vi "FPGA Main.vi"(8 "Read":bool) -> (4 "Element in Buffer":u32[](array[numeric])=[189, 189, 189, 189])   [LabVIEW 2011]
uses:
  <vilib>/rvi/eio/common/nirviEmuTemplateMethod_errors.vi
  <vilib>/rvi/DataTransferAndStorage/Container/Common/niFpgaContainerExecOnDevCompGetState.vi
  <vilib>/rvi/FIFO/Fifo_Resource/nirvififoEmulationSetSize.vi
  <vilib>/rvi/DataTransferAndStorage/Container/Common/niFpgaContainerGetUniqueNameForEmu.vi
  <vilib>/rvi/interface/RandomDataEmulation/nirviRandomDataFPGAFIFO.vi
  <vilib>/rvi/interface/RandomDataEmulation/niFpgaRandomDataHandleErrors.vi
  <vilib>/rvi/eio/common/nirviEmuReportErrorAndStop.vi
  Global_Read.vi
  <vilib>/eio/EIONode/EIONode.xnode
  <vilib>/rvi/DataTransferAndStorage/Container/XNode/niFpgaContainer.xnode
  <vilib>/rvi/FIFO/Fifo_Resource/niFpgaFifoEmulationRefIn.vi
panel:
  out "Beat":bool=TRUE
  in  "Edge":bool
  in  "Buffer#4":i32
  in  "Buffer#3":i32
  in  "Buffer#2":i32
  in  "Buffer#1":i32
  in  "Port Settings - 4 Chan":T1(array[cluster])=[{"Data Bit(8)"=8, "Stop Bit"=1, "Baud Rate"=9600, "Invert Polarity?"=TRUE, " Mode"=FALSE}, {"Data Bit(8)"=0, "Stop Bit"=0, "Baud Rate"=0, "Invert Polarity?"=FALSE, " Mode"=FALSE}, {"Data Bit(8)"=0, "Stop Bit"=0, "Baud Rate"=0, "Invert Polarity?"=FALSE, " Mode"=FALSE}, {"Data Bit(8)"=0, "Stop Bit"=0, "Baud Rate"=0, "Invert Polarity?"=FALSE, " Mode"=FALSE}] {"Stop Bit" items=["1.0"=10, "1.5"=15, "2.0"=20]}
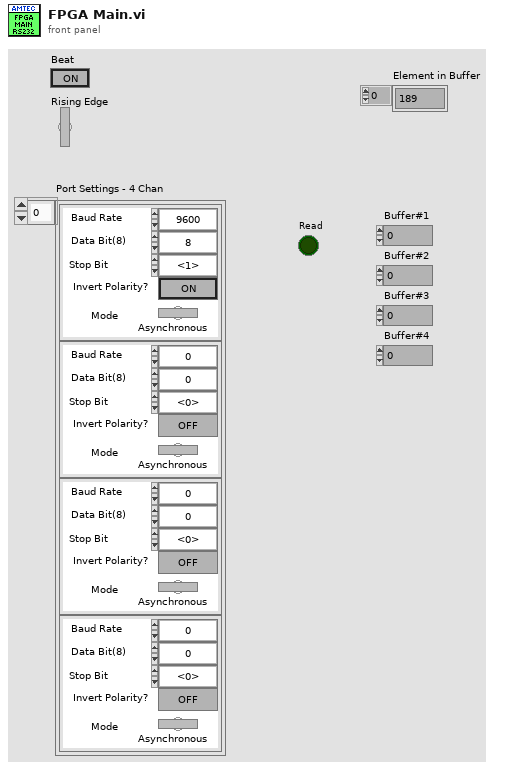
[diagram p1: front panel]
types:
  T1 = cluster{"Data Bit(8)":i32, "Stop Bit":u16, "Baud Rate":u32, "Invert Polarity?":bool, " Mode":bool}[]
  T2 = cluster{"Data Bit(8)":i32, "Stop Bit":u16, "Baud Rate":u32, "Invert Polarity?":bool, " Mode":bool}
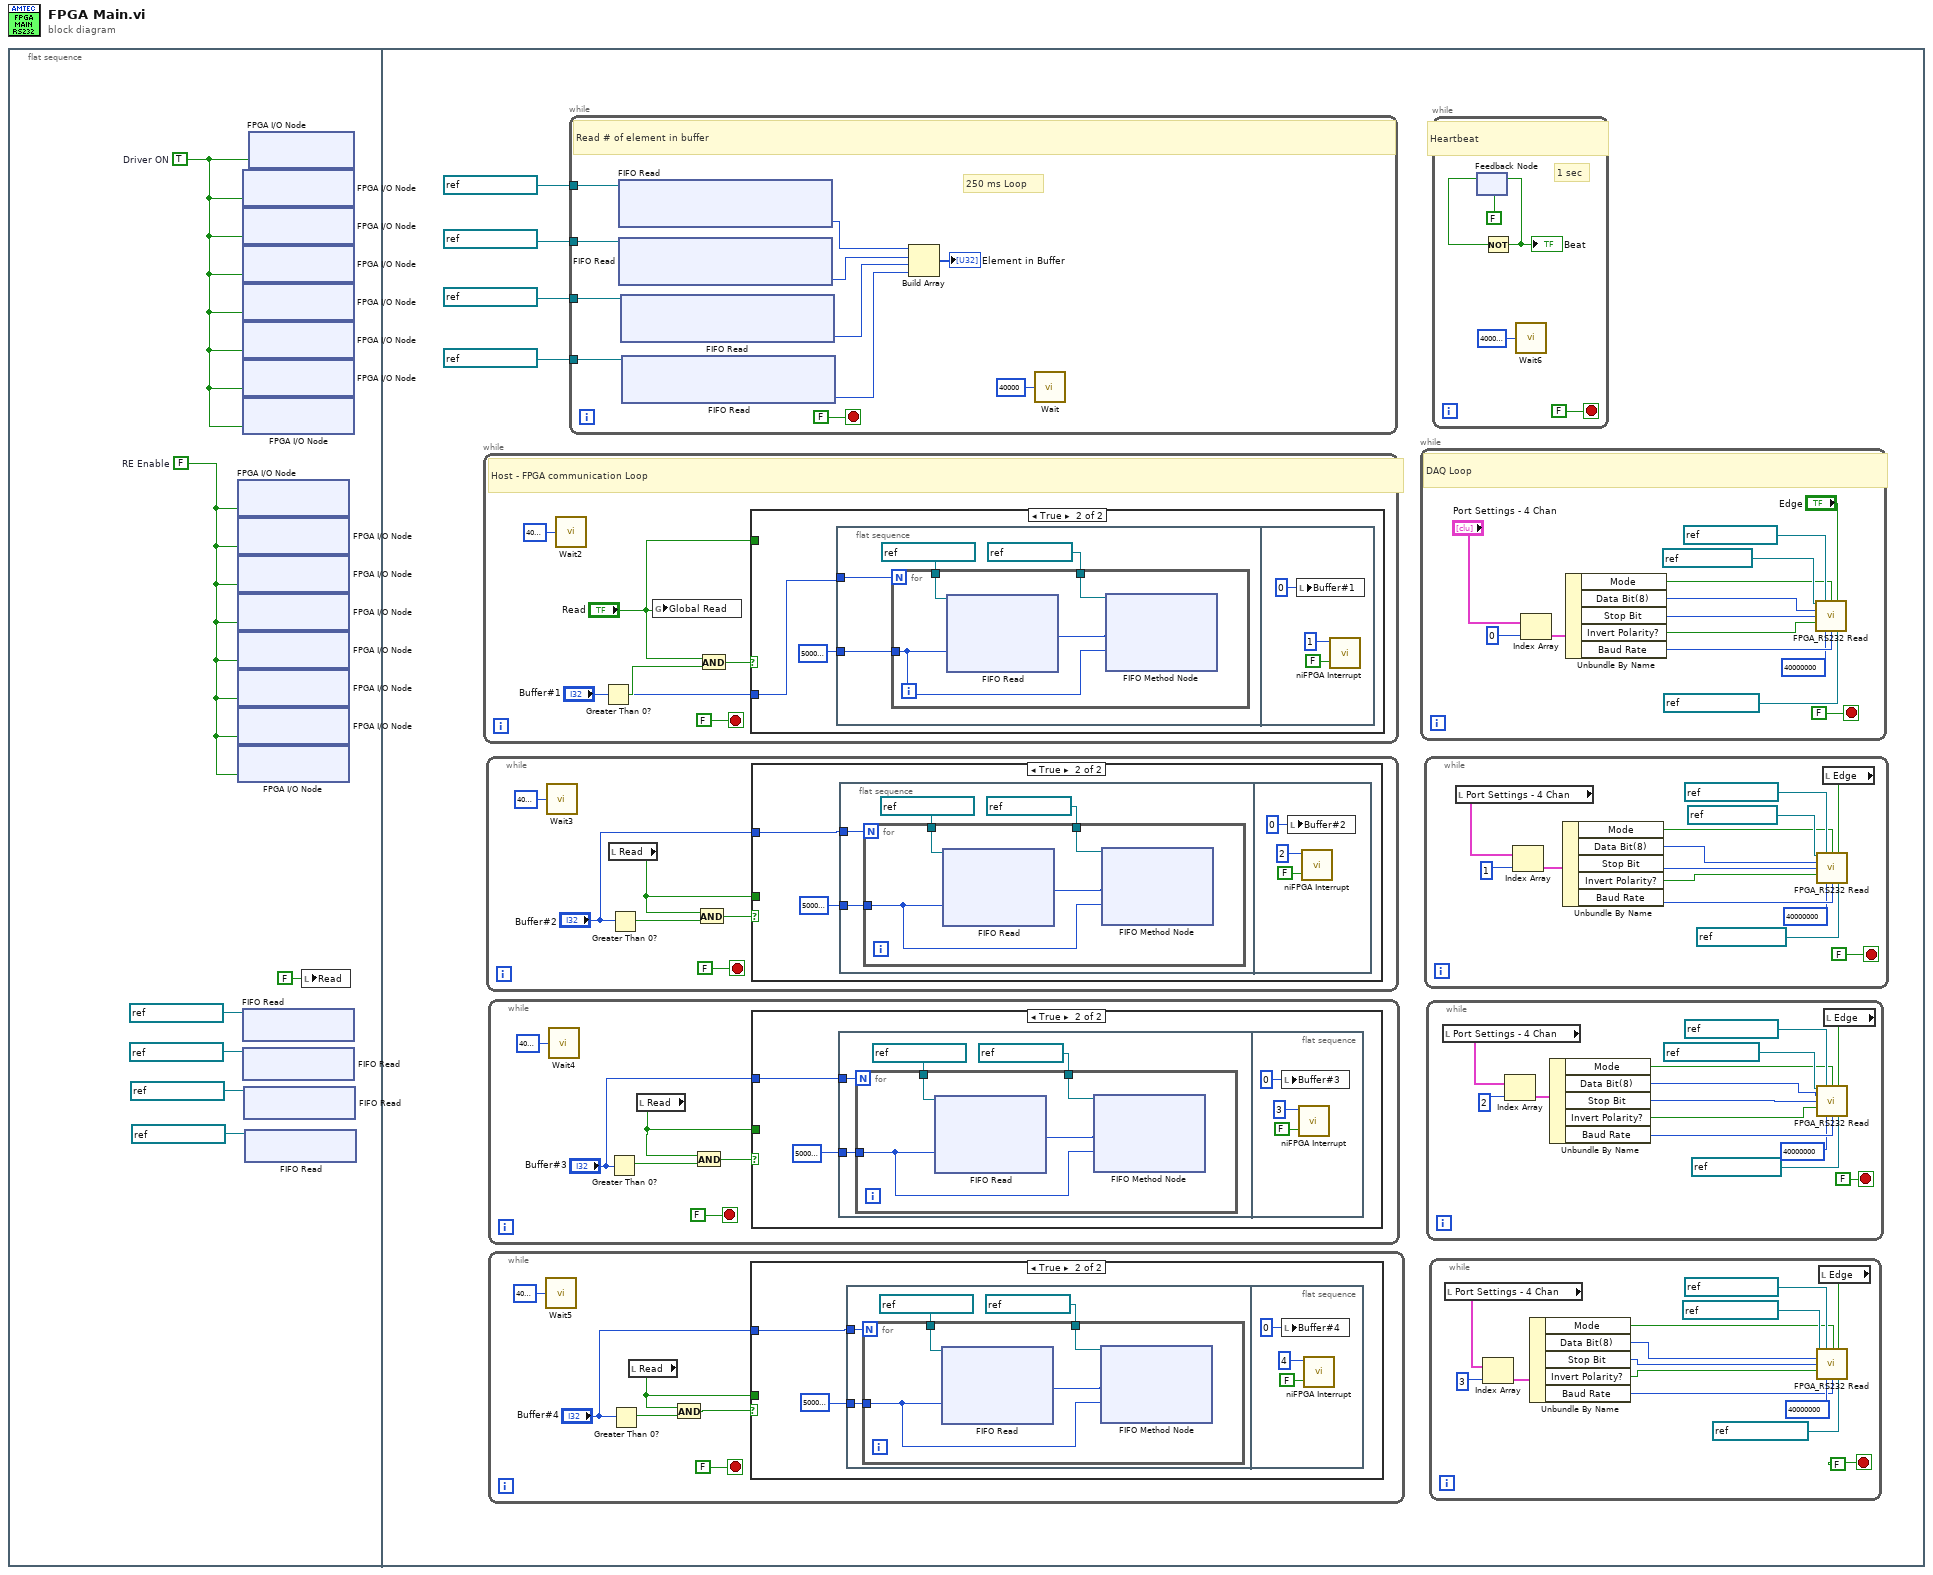
[diagram p0: block diagram]
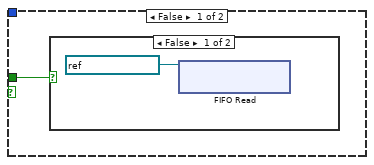
[diagram p2: hidden frame]
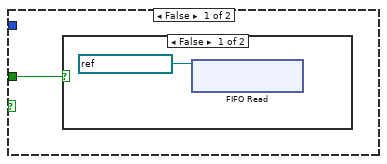
[diagram p4: hidden frame]
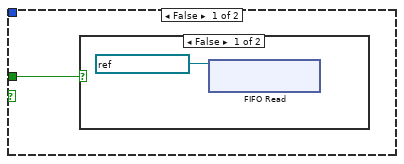
[diagram p6: hidden frame]
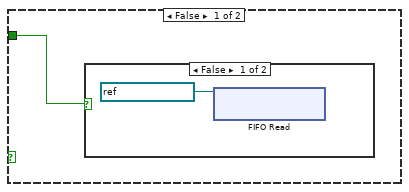
[diagram p8: hidden frame]
diagram:
  n1 = flat-sequence {
    frame #0 {
      w2 = TRUE  # Driver ON
      w1 = FALSE  # RE Enable
      n2 = xnode "FPGA I/O Node"("JAGM/DIO32"=w1) -> ()  [unwired: 1 in, 1 out]
      n3 = xnode "FPGA I/O Node"("JAGM/DIO41"=w1) -> ()  [unwired: 1 in, 1 out]
      n4 = xnode "FPGA I/O Node"("JAGM/DIO47"=w1) -> ()  [unwired: 1 in, 1 out]
      n5 = xnode "FPGA I/O Node"("JAGM/DIO54"=w1) -> ()  [unwired: 1 in, 1 out]
      n6 = xnode "FPGA I/O Node"("JAGM/DIO50"=w1) -> ()  [unwired: 1 in, 1 out]
      n7 = xnode "FPGA I/O Node"("JAGM/DIO37"=w1) -> ()  [unwired: 1 in, 1 out]
      n8 = xnode "FPGA I/O Node"("JAGM/DIO45"=w1) -> ()  [unwired: 1 in, 1 out]
      n9 = xnode "FPGA I/O Node"("JAGM/DIO27"=w1) -> ()  [unwired: 1 in, 1 out]
      n10 = xnode "FPGA I/O Node"("JAGM/DIO38"=w2) -> ()  [unwired: 1 in, 1 out]
      n11 = xnode "FPGA I/O Node"("JAGM/DIO15"=w2) -> ()  [unwired: 1 in, 1 out]
      n12 = xnode "FPGA I/O Node"("JAGM/DIO55"=w2) -> ()  [unwired: 1 in, 1 out]
      n13 = xnode "FPGA I/O Node"("JAGM/DIO52"=w2) -> ()  [unwired: 1 in, 1 out]
      n14 = xnode "FPGA I/O Node"("JAGM/DIO35"=w2) -> ()  [unwired: 1 in, 1 out]
      n15 = xnode "FPGA I/O Node"("JAGM/DIO43"=w2) -> ()  [unwired: 1 in, 1 out]
      n16 = xnode "FPGA I/O Node"("JAGM/DIO60"=w2) -> ()  [unwired: 1 in, 1 out]
      n17 = xnode ("FIFO Read")("FIFO In"=refnum<k21> "FIFO_Chan 1") -> ()  [unwired: 1 out]
      n18 = xnode ("FIFO Read")("FIFO In"=refnum<k21> "FIFO_Chan 2") -> ()  [unwired: 1 out]
      n19 = xnode ("FIFO Read")("FIFO In"=refnum<k21> "FIFO_Chan 3") -> ()  [unwired: 1 out]
      n20 = xnode ("FIFO Read")("FIFO In"=refnum<k21> "FIFO_Chan 4") -> ()  [unwired: 1 out]
      n21 = xnode "FPGA I/O Node"("JAGM/DIO0"=w2) -> ()  [unwired: 1 in, 1 out]
      n22 = local write "Read"(FALSE ("Read")) -> ()
    }
    frame #1 {
      n23 = while {
        stop <- FALSE stop-if-true
        # "Host - FPGA communication Loop"
        n24 = call "Wait2"("Count(Ticks)"=u32 4000000) -> ()  [unwired: 1 out]
        n25 = Greater Than 0?(x="Buffer#1") -> (x > 0?=w85:bool)
        n26 = global write "Global_Read.vi" "Global Read"("Read") -> ()
        n27 = And(x="Read", y=w85) -> (x .and. y?=w84:bool)
        n28 = case shown="True" w84 {
          tunnel: "Buffer#1" -> [_ w89]
          tunnel: "Read" -> [w86 _]
          frame False {
            n29 = case shown="False" w86 {
              frame False {
                n30 = xnode ("FIFO Read")("FIFO In"=refnum<k21> "FIFO_Chan 1") -> ()  [unwired: 1 out]
              }
              frame True {
              }
            }
          }
          frame True {
            n31 = flat-sequence {
              tunnel: w89 -> [w93]
              tunnel: u32 50000000 ("Count(Ticks)") -> [w92]
              frame #0 {
                n32 = for {
                  N: w93 -> [_]
                  tunnel: w92 -> [w95]
                  tunnel: refnum<k21> "H-T FIFO 1" ("FIFO In") -> [w97]
                  tunnel: refnum<k21> "FIFO_Chan 1" ("FIFO In") -> [w94]
                  n33 = xnode ("FIFO Read")("Timeout"=w95, "FIFO In"=w94) -> ("Element"=w96:u8)  [unwired: 2 out]
                  n34 = xnode ("FIFO Method Node")("Element"=w96, "Timeout"=w95, "FIFO In"=w97) -> ()  [unwired: 2 out]
                }
              }
              frame #1 {
                n35 = local write "Buffer#1"(0 ("Buffer#4")) -> ()
                n36 = call <vilib>:"niFPGA Interrupt.vi"("Wait Until Cleared"=FALSE, "IRQ Number"=u8 1 ("IRQBit")) -> ()  [unwired: 1 in]
              }
            }
          }
        }
      }
      n37 = while {
        stop <- FALSE stop-if-true
        n38 = call "Wait3"("Count(Ticks)"=u32 4000000) -> ()  [unwired: 1 out]
        n39 = local read "Read"() -> (w60:bool)
        n40 = Greater Than 0?(x="Buffer#2") -> (x > 0?=w63:bool)
        n41 = And(x=w60, y=w63) -> (x .and. y?=w64:bool)
        n42 = case shown="True" w64 {
          tunnel: "Buffer#2" -> [_ w68]
          tunnel: w60 -> [w65 _]
          frame False {
            n43 = case shown="False" w65 {
              frame False {
                n44 = xnode ("FIFO Read")("FIFO In"=refnum<k21> "FIFO_Chan 2") -> ()  [unwired: 1 out]
              }
              frame True {
              }
            }
          }
          frame True {
            n45 = flat-sequence {
              tunnel: w68 -> [w72]
              tunnel: u32 50000000 ("Count(Ticks)") -> [w71]
              frame #0 {
                n46 = for {
                  N: w72 -> [_]
                  tunnel: w71 -> [w74]
                  tunnel: refnum<k21> "H-T FIFO 2" ("FIFO In") -> [w76]
                  tunnel: refnum<k21> "FIFO_Chan 2" ("FIFO In") -> [w73]
                  n47 = xnode ("FIFO Read")("Timeout"=w74, "FIFO In"=w73) -> ("Element"=w75:u8)  [unwired: 2 out]
                  n48 = xnode ("FIFO Method Node")("Element"=w75, "Timeout"=w74, "FIFO In"=w76) -> ()  [unwired: 2 out]
                }
              }
              frame #1 {
                n49 = local write "Buffer#2"(0 ("Buffer#4")) -> ()
                n50 = call <vilib>:"niFPGA Interrupt.vi"("Wait Until Cleared"=FALSE, "IRQ Number"=u8 2 ("IRQBit")) -> ()  [unwired: 1 in]
              }
            }
          }
        }
      }
      n51 = while {
        stop <- FALSE stop-if-true
        n52 = call "Wait4"("Count(Ticks)"=u32 4000000) -> ()  [unwired: 1 out]
        n53 = Greater Than 0?(x="Buffer#3") -> (x > 0?=w42:bool)
        n54 = local read "Read"() -> (w39:bool)
        n55 = And(x=w39, y=w42) -> (x .and. y?=w43:bool)
        n56 = case shown="True" w43 {
          tunnel: "Buffer#3" -> [_ w47]
          tunnel: w39 -> [w44 _]
          frame False {
            n57 = case shown="False" w44 {
              frame False {
                n58 = xnode ("FIFO Read")("FIFO In"=refnum<k21> "FIFO_Chan 3") -> ()  [unwired: 1 out]
              }
              frame True {
              }
            }
          }
          frame True {
            n59 = flat-sequence {
              tunnel: w47 -> [w51]
              tunnel: u32 50000000 ("Count(Ticks)") -> [w50]
              frame #0 {
                n60 = for {
                  N: w51 -> [_]
                  tunnel: w50 -> [w53]
                  tunnel: refnum<k21> "H-T FIFO 3" ("FIFO In") -> [w55]
                  tunnel: refnum<k21> "FIFO_Chan 3" ("FIFO In") -> [w52]
                  n61 = xnode ("FIFO Read")("Timeout"=w53, "FIFO In"=w52) -> ("Element"=w54:u8)  [unwired: 2 out]
                  n62 = xnode ("FIFO Method Node")("Element"=w54, "Timeout"=w53, "FIFO In"=w55) -> ()  [unwired: 2 out]
                }
              }
              frame #1 {
                n63 = local write "Buffer#3"(0 ("Buffer#4")) -> ()
                n64 = call <vilib>:"niFPGA Interrupt.vi"("Wait Until Cleared"=FALSE, "IRQ Number"=u8 3 ("IRQBit")) -> ()  [unwired: 1 in]
              }
            }
          }
        }
      }
      n65 = while {
        stop <- FALSE stop-if-true
        n66 = call "Wait5"("Count(Ticks)"=u32 4000000) -> ()  [unwired: 1 out]
        n67 = Greater Than 0?(x="Buffer#4") -> (x > 0?=w22:bool)
        n68 = local read "Read"() -> (w18:bool)
        n69 = And(x=w18, y=w22) -> (x .and. y?=w21:bool)
        n70 = case shown="True" w21 {
          tunnel: "Buffer#4" -> [_ w26]
          tunnel: w18 -> [w23 _]
          frame False {
            n71 = case shown="False" w23 {
              frame False {
                n72 = xnode ("FIFO Read")("FIFO In"=refnum<k21> "FIFO_Chan 4") -> ()  [unwired: 1 out]
              }
              frame True {
              }
            }
          }
          frame True {
            n73 = flat-sequence {
              tunnel: w26 -> [w30]
              tunnel: u32 50000000 ("Count(Ticks)") -> [w29]
              frame #0 {
                n74 = for {
                  N: w30 -> [_]
                  tunnel: w29 -> [w32]
                  tunnel: refnum<k21> "H-T FIFO 4" ("FIFO In") -> [w34]
                  tunnel: refnum<k21> "FIFO_Chan 4" ("FIFO In") -> [w31]
                  n75 = xnode ("FIFO Read")("Timeout"=w32, "FIFO In"=w31) -> ("Element"=w33:u8)  [unwired: 2 out]
                  n76 = xnode ("FIFO Method Node")("Element"=w33, "Timeout"=w32, "FIFO In"=w34) -> ()  [unwired: 2 out]
                }
              }
              frame #1 {
                n77 = local write "Buffer#4"(0 ("Buffer#4")) -> ()
                n78 = call <vilib>:"niFPGA Interrupt.vi"("Wait Until Cleared"=FALSE, "IRQ Number"=u8 4 ("IRQBit")) -> ()  [unwired: 1 in]
              }
            }
          }
        }
      }
      n79 = while {
        tunnel: refnum<k21> "FIFO_Chan 1" ("FIFO In") -> [w167]
        tunnel: refnum<k21> "FIFO_Chan 2" ("FIFO In") -> [w166]
        tunnel: refnum<k21> "FIFO_Chan 3" ("FIFO In") -> [w165]
        tunnel: refnum<k21> "FIFO_Chan 4" ("FIFO In") -> [w164]
        stop <- FALSE stop-if-true
        # "250 ms Loop"
        # "Read # of element in buffer"
        n80 = xnode ("FIFO Read")("FIFO In"=w167) -> ("Number of Elements to Read"=w162:u32)  [unwired: 1 out]
        n81 = xnode ("FIFO Read")("FIFO In"=w166) -> ("Number of Elements to Read"=w161:u32)  [unwired: 1 out]
        n82 = xnode ("FIFO Read")("FIFO In"=w165) -> ("Number of Elements to Read"=w160:u32)  [unwired: 1 out]
        n83 = xnode ("FIFO Read")("FIFO In"=w164) -> ("Number of Elements to Read"=w159:u32)  [unwired: 1 out]
        n84 = Build Array(w162, w161, w160, w159) -> (→"Element in Buffer":u32[])
        n85 = call "Wait"("Count(Ticks)"=u32 40000) -> ()  [unwired: 1 out]
      }
      n86 = while {
        stop <- FALSE stop-if-true
        # "DAQ Loop"
        n87 = Index Array(array="Port Settings - 4 Chan", index=0) -> (element=w154:T2)
        n88 = Unbundle By Name(w154) -> ("Mode"=w144:bool, "Data Bit(8)"=w151:i32, "Stop Bit"=w150:u16, "Invert Polarity?"=w148:bool, "Baud Rate"=w149:u32)
        n89 = call "FPGA_RS232 Read.vi"("Receive"=refnum<k21> "JAGM/DIO2", "FIFO In"=refnum<k21> "FIFO_Chan 1", "Mode"=w144, "Edge"="Edge", "data bits (8)"=w151, "Stop Bit"=w150, "Invert Polarity?"=w148, "Clock Rate"=u32 40000000, "baud rate"=w149, "Clk"=refnum<k21> "JAGM/DIO16") -> ()  [unwired: 5 in, 1 out]
      }
      n90 = while {
        stop <- FALSE stop-if-true
        n91 = local read "Port Settings - 4 Chan"() -> (w130:T1)
        n92 = Index Array(array=w130, index=1) -> (element=w141:T2)
        n93 = Unbundle By Name(w141) -> ("Mode"=w132:bool, "Data Bit(8)"=w138:i32, "Stop Bit"=w137:u16, "Invert Polarity?"=w136:bool, "Baud Rate"=w135:u32)
        n94 = local read "Edge"() -> (w129:bool)
        n95 = call "FPGA_RS232 Read.vi"("Receive"=refnum<k21> "JAGM/DIO6", "FIFO In"=refnum<k21> "FIFO_Chan 2", "Mode"=w132, "Edge"=w129, "data bits (8)"=w138, "Stop Bit"=w137, "Invert Polarity?"=w136, "Clock Rate"=u32 40000000, "baud rate"=w135, "Clk"=refnum<k21> "JAGM/DIO4") -> ()  [unwired: 5 in, 1 out]
      }
      n96 = while {
        stop <- FALSE stop-if-true
        n97 = local read "Port Settings - 4 Chan"() -> (w116:T1)
        n98 = Index Array(array=w116, index=2) -> (element=w127:T2)
        n99 = Unbundle By Name(w127) -> ("Mode"=w118:bool, "Data Bit(8)"=w124:i32, "Stop Bit"=w123:u16, "Invert Polarity?"=w122:bool, "Baud Rate"=w121:u32)
        n100 = local read "Edge"() -> (w115:bool)
        n101 = call "FPGA_RS232 Read.vi"("Receive"=refnum<k21> "JAGM/DIO10", "FIFO In"=refnum<k21> "FIFO_Chan 3", "Mode"=w118, "Edge"=w115, "data bits (8)"=w124, "Stop Bit"=w123, "Invert Polarity?"=w122, "Clock Rate"=u32 40000000, "baud rate"=w121, "Clk"=refnum<k21> "JAGM/DIO8") -> ()  [unwired: 5 in, 1 out]
      }
      n102 = while {
        stop <- FALSE stop-if-true
        n103 = local read "Port Settings - 4 Chan"() -> (w104:T1)
        n104 = Index Array(array=w104, index=3) -> (element=w113:T2)
        n105 = Unbundle By Name(w113) -> ("Mode"=w106:bool, "Data Bit(8)"=w110:i32, "Stop Bit"=w109:u16, "Invert Polarity?"=w108:bool, "Baud Rate"=w101:u32)
        n106 = local read "Edge"() -> (w103:bool)
        n107 = call "FPGA_RS232 Read.vi"("Receive"=refnum<k21> "JAGM/DIO14", "FIFO In"=refnum<k21> "FIFO_Chan 4", "Mode"=w106, "Edge"=w103, "data bits (8)"=w110, "Stop Bit"=w109, "Invert Polarity?"=w108, "Clock Rate"=u32 40000000, "baud rate"=w101, "Clk"=refnum<k21> "JAGM/DIO12") -> ()  [unwired: 5 in, 1 out]
      }
      n108 = while {
        stop <- FALSE stop-if-true
        # "1 sec"
        # "Heartbeat"
        n109 = feedback #1(FALSE) -> (w14:bool)
        n110 = Not(x=w14) -> (.not. x?=w16:bool)
        "Beat" <- w16
        n111 = feedback-in #1(w16) -> ()
        n112 = call "Wait6"("Count(Ticks)"=u32 40000000) -> ()  [unwired: 1 out]
      }
    }
  }
